vi "Ungueltiger Messwert.vi"(8 "Stöung Messgerät":bool, 10 "Messwert":sgl) -> (2 "Messwert String":string)   [LabVIEW 2020, in "AK-Schnittstelle.lvlib"]
uses:
  AK-Schnittstelle.lvlib
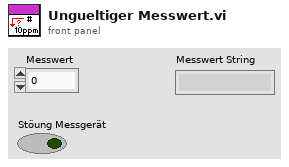
[diagram p1: front panel]
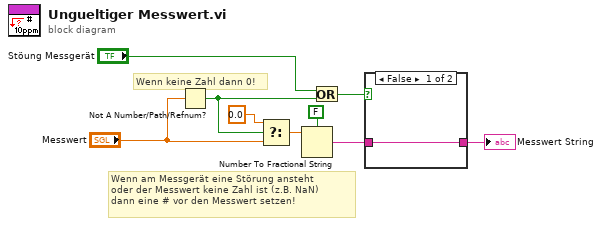
[diagram p0: block diagram]
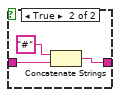
[diagram p2: hidden frame]
diagram:
  # "Wenn keine Zahl dann 0!"
  # "Wenn am Messgerät eine Störung ansteht \noder der Messwert keine Zahl ist (z.B. NaN) \ndann eine # vor den Messwert setzen!"
  n1 = Not A Number/Path/Refnum?(number/path/refnum="Messwert") -> (NaN/Path/Refnum?=w9:bool)
  n2 = Select(t=0.0, s=w9, f="Messwert") -> (s? t:f=w5:dbl)
  n3 = Number To Fractional String(use system decimal point (T)=FALSE ("Systemdezimalzeichen verwenden (T)"), number=w5) -> (F-format string=w4:string)  [unwired: 2 in]
  n4 = Or(x="Stöung Messgerät", y=w9) -> (x .or. y?=w6:bool)
  n5 = case shown="False" w6 {
    tunnel: w4 -> [w10 w13]
    tunnel: [w10 w11] -> w3
    frame False {
    }
    frame True {
      n6 = Concatenate Strings("#" ("String"), w13) -> (w11:string)
    }
  }
  "Messwert String" <- w3
